vi "Start Client.vi"(6 "timeout ms (5)":i32=5, 7 "JSON {\"verbose\":false}":string="{\"verbose\":false}", 8 "error in":errorcluster {"code" format="Error %.0f"}, 9 "bytes to read (1024)":i32=1024, 10 "port (4222)":u16=4222, 11 "address":string="localhost") -> (0 "error out":errorcluster {"code" format="Error %.0f"}, 3 "NATS Client out":refnum<class "NATS Client.lvclass">)   [LabVIEW 2020, in "NATS Client.lvlib" / "NATS Client.lvclass"]
doc: "Starts the Client asynchronous daemon. The daemon must be started to use other NATS Client.lvclass methods."
uses:
  NATS Client.lvclass
  NATS Subscription/NATS Subscription.lvclass
  NATS Client.lvclass/NATS Client.ctl
  Async.vi
  subscription actions.ctl
  subscription queue.ctl
  <vilib>/NATS/NATS Core/NATS Core.lvlib
  Reconnect Parameters.ctl
  Subscription Map.ctl
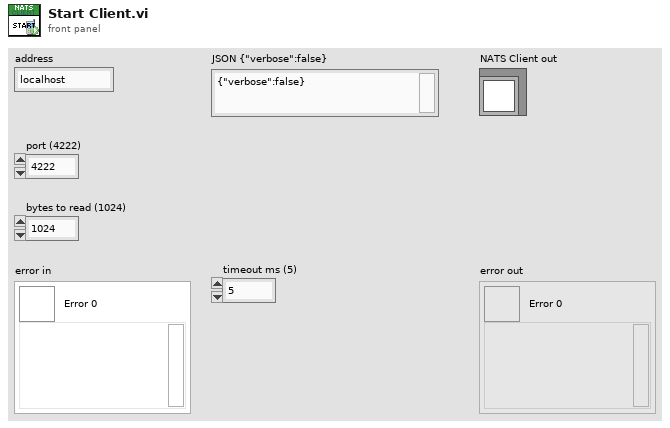
[diagram p1: front panel]
types:
  T1 = typedef "NATS Client.lvlib/NATS Client.lvclass/Subscription Map.ctl" = map{string, refnum<class "NATS Subscription.lvclass">}
  T2 = typedef "NATS Client.lvlib/NATS Client.lvclass/Reconnect Parameters.ctl" = cluster{"IP Address":string, "JSON":string, "bytes to read (1024)":i32, "timeout ms (5)":i32, "port (4222)":u16}
  T3 = typedef "NATS Client.lvlib/NATS Client.lvclass/subscription queue.ctl" = cluster{"action":T4, "subscription":refnum<class "NATS Subscription.lvclass">}
  T4 = typedef "NATS Client.lvlib/NATS Client.lvclass/subscription actions.ctl" = enum16{"sub", "unsub"}
  T5 = typedef "NATS Core.lvlib/nats connection.ctl" = cluster{"connection ID":refnum<k5>, "server INFO":string, "timeout ms":i32, "verbose?":bool, "server headers?":bool, "client headers?":bool}
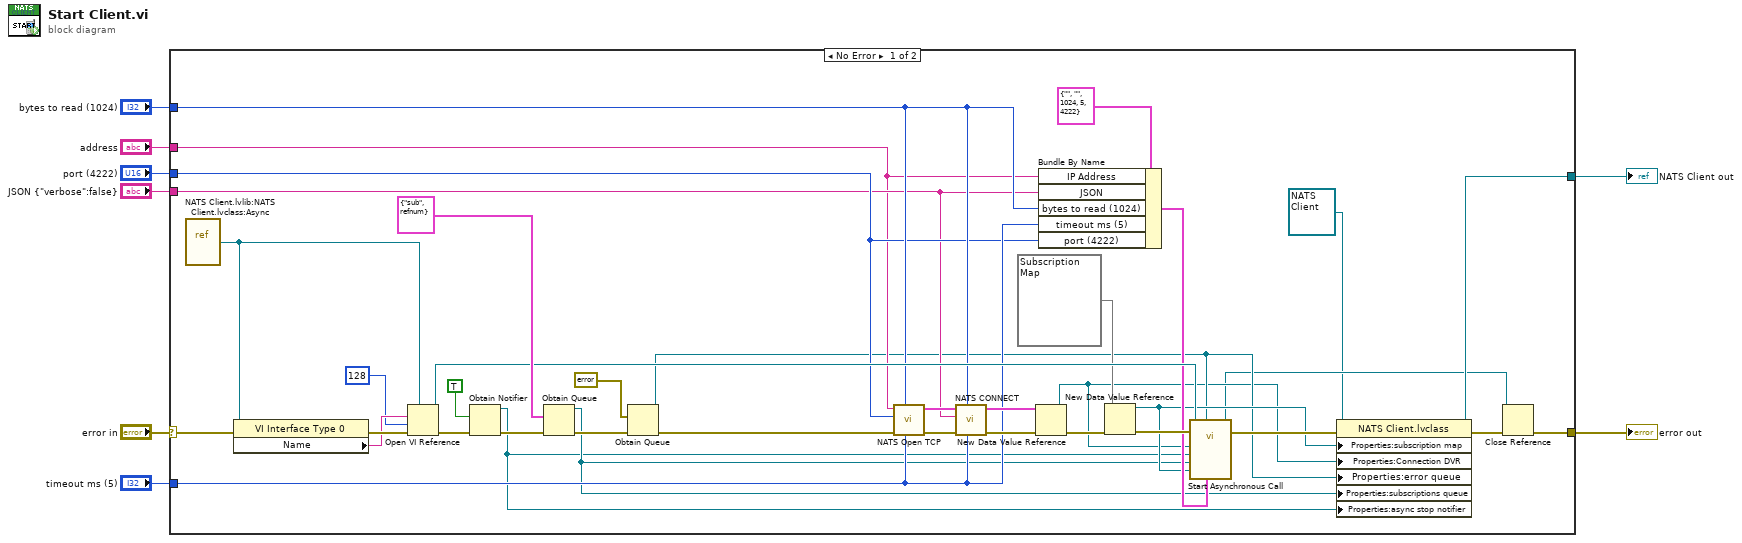
[diagram p0: block diagram]
diagram:
  n1 = case shown="No Error" "error in" {
    selector: "error in" -> [w35 w47]
    tunnel: [w14 w47] -> w7
    tunnel: [w42 _] -> w6
    tunnel: "address" -> [w24 _]
    tunnel: "bytes to read (1024)" -> [w28 _]
    tunnel: "timeout ms (5)" -> [w27 _]
    tunnel: "port (4222)" -> [w26 _]
    tunnel: "JSON {\"verbose\":false}" -> [w25 _]
    frame No Error {
      n2 = vi-ref "NATS Client.lvlib:NATS Client.lvclass:Async.vi"() -> (w36:refnum<vi>)
      n3 = property class="VI Interface Type 0"(reference=w36, error in=w35) -> (error out=w34:errorcluster, "Name"=w33:string)  [unwired: 1 out]
      n4 = Open VI Reference(type specifier VI Refnum (for type only)=w36, vi path=w33, options=128, error in (no error)=w34) -> (vi reference=w37:refnum<vi>, error out=w38:errorcluster)  [unwired: 2 in]
      n5 = Obtain Notifier(notification data type=TRUE ("create if not found?"), error in (no error)=w38) -> (notifier out=w10:refnum<notifier>, error out=w44:errorcluster)  [unwired: 2 in, 1 out]
      n6 = Obtain Queue(element data type=T3 {"action"=enum."sub", "subscription"=refnum} ("subscription queue"), error in (no error)=w44) -> (queue out=w11:refnum<queue>, error out=w46:errorcluster)  [unwired: 3 in, 1 out]
      n7 = Obtain Queue(element data type=errorcluster {"status"=FALSE, "code"=0, "source"=""} ("error out"), error in (no error)=w46) -> (queue out=w16:refnum<queue>, error out=w23:errorcluster)  [unwired: 3 in, 1 out]
      n8 = call <vilib>:"NATS Open TCP.vi"("timeout ms (5000)"=w27, "bytes to read (1024)"=w28, "error in"=w23, "port (4222)"=w26, "address"=w24) -> ("error out"=w43:errorcluster, "nats connection"=w40:T5)  [unwired: 3 in, 2 out]
      n9 = call <vilib>:"NATS CONNECT.vi"("timeout ms (conn default)"=w27, "bytes to read (1024)"=w28, "error in"=w43, "JSON"=w25, "nats connection in"=w40) -> ("error out"=w31:errorcluster, "nats connection out"=w32:T5)  [unwired: 4 in, 1 out]
      n10 = New Data Value Reference(data value=w32, error in=w31) -> (data value reference=w15:refnum<data-value>, error out=w20:errorcluster)
      n11 = Bundle By Name(cluster=T2 {"IP Address"="", "JSON"="", "bytes to read (1024)"=1024, "timeout ms (5)"=5, "port (4222)"=4222}, "IP Address"=w24, "JSON"=w25, "bytes to read (1024)"=w28, "timeout ms (5)"=w27, "port (4222)"=w26) -> (w18:T2)
      n12 = New Data Value Reference(data value=T1 {} ("subs in"), error in=w20) -> (data value reference=w17:refnum<data-value>, error out=w19:errorcluster)
      n13 = call-by-ref "Start Asynchronous Call"(reference=w37, error in=w19, "Reconnect Parameters"=w18, "error queue"=w16, "sub map"=w17, "subscriptions queue"=w11, "async stop notifier"=w10, "NATS Connection"=w15) -> (reference out=w13:refnum<vi>, error out=w30:errorcluster)  [unwired: 6 in]
      n14 = property class="NATS Client.lvclass"(reference=refnum<class "NATS Client.lvclass"> refnum ("NATS Client out"), error in=w30, "Properties:subscription map"=w17, "Properties:Connection DVR"=w15, "Properties:error queue"=w16, "Properties:subscriptions queue"=w11, "Properties:async stop notifier"=w10) -> (reference out=w42:refnum<class "NATS Client.lvclass">, error out=w45:errorcluster)
      n15 = Close Reference(reference=w13, error in (no error)=w45) -> (error out=w14:errorcluster)
    }
    frame Error {
    }
  }
  "error out" <- w7
  "NATS Client out" <- w6
